vi "Sensor_limit_H.vi"(9 "Off H":dbl, 10 "PV":dbl, 11 "Limit H":dbl) -> (1 "Off":bool, 2 "On":bool, 3 "NaN":bool)   [LabVIEW 2019, in "Inputs.lvlib"]
uses:
  Inputs.lvlib
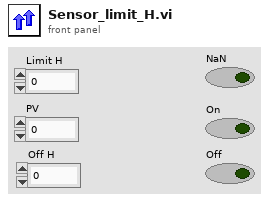
[diagram p1: front panel]
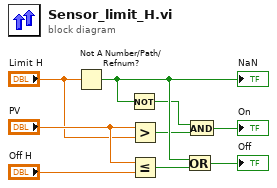
[diagram p0: block diagram]
diagram:
  n1 = Not A Number/Path/Refnum?(number/path/refnum="Limit H") -> (NaN/Path/Refnum?=w7:bool)
  "NaN" <- w7
  n2 = Not(x=w7) -> (.not. x?=w5:bool)
  n3 = Greater?(x="PV", y="Limit H") -> (0:w2:bool)
  n4 = Less Or Equal?(x="PV", y="Off H") -> (x <= y?=w3:bool)
  n5 = Or(x=w7, y=w3) -> (x .or. y?=→"Off":bool)
  n6 = And(x=w5, y=w2) -> (x .and. y?=→"On":bool)
